vi "SaveData_Rf.vi"(8 "error in (no error)":errorcluster, 11 "Data In":T1) -> (0 "error out":errorcluster, 3 "Data Out":T1)   [LabVIEW 2014]
uses:
  controls/Data.ctl
  <vilib>/Utility/file.llb/Write To Spreadsheet File (string).vi
panel:
  # "日期"
  # "機種名稱"
  # "機種代號"
  # "商品條碼"
  # "台"
  # "OK"
  # "NG"
  # "台"
  # "總計"
  # "台"
  # "日期"
  # "機種名稱"
  # "機種代號"
  # "商品條碼"
  # "台"
  # "OK"
  # "NG"
  # "台"
  # "總計"
  # "台"
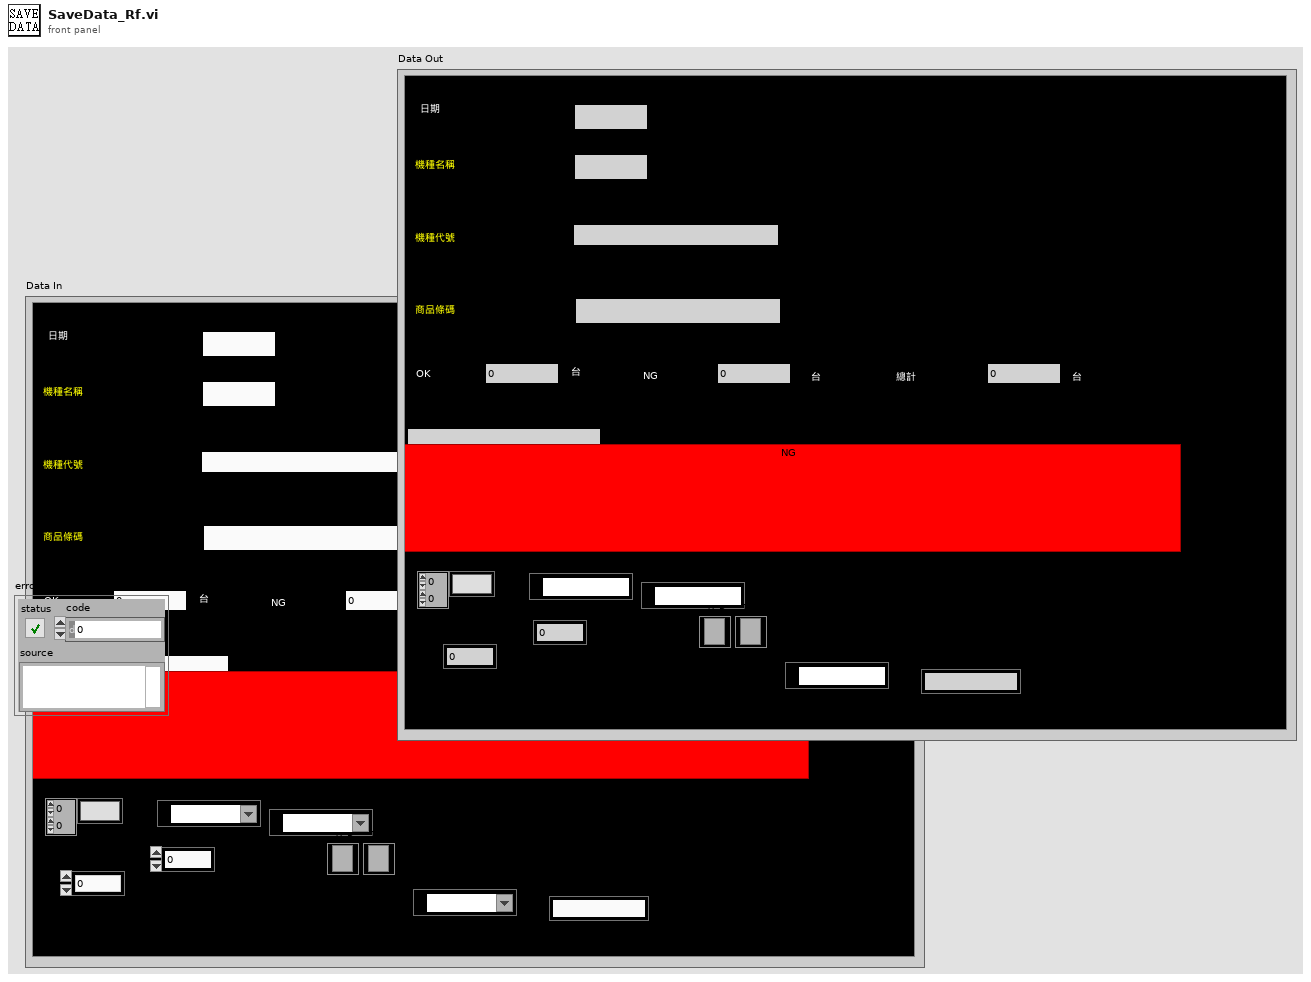
[diagram p1: front panel]
types:
  T1 = typedef "Data.ctl" = cluster{"Date":string, "BarCode1":string, "BarCode2":string, "BarCode3":string, "Message":string, "OK Count":u16, "NG Count":u16, "Total Count":u16, "ModelData":string[][], "OK&NG":bool, "COM1":refnum<visa-resource-name>, "COM2":refnum<visa-resource-name>, "IO":i32, "Time":u32, "TCP":refnum<k5>, "TCP 2":refnum<k5>, "COM3":refnum<visa-resource-name>, "CheckPars":string}
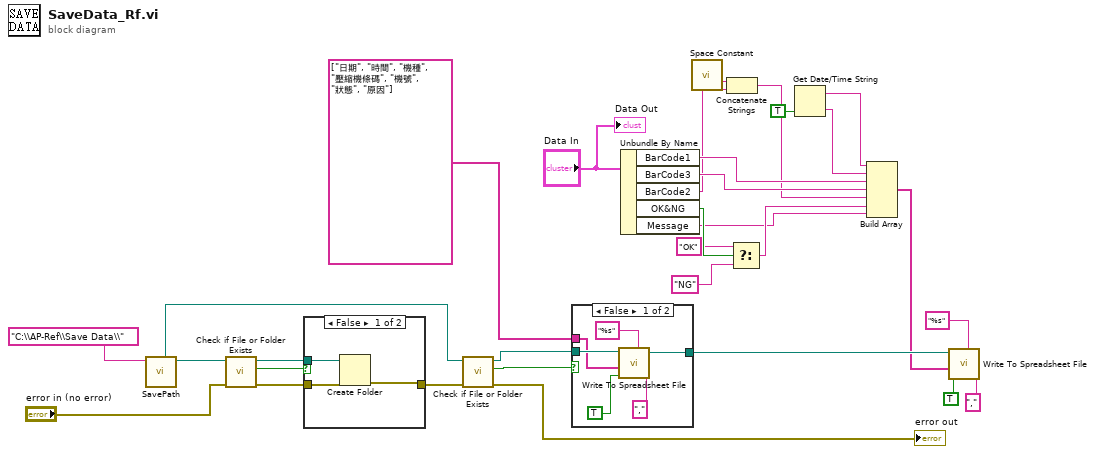
[diagram p0: block diagram]
diagram:
  n1 = call "SavePath.vi"("Path In"="C:\\AP-Ref\\Save Data\\") -> ("Folder Path"=w28:path, "File Path"=w26:path)  [unwired: 9 in]
  n2 = call <vilib>:"Check if File or Folder Exists.vi"("error in (no error)"="error in (no error)", "path"=w28) -> ("error out"=w25:errorcluster, "file or folder exists?"=w27:bool, "dup path"=w23:path)  [unwired: 7 in]
  n3 = case shown="False" w27 {
    tunnel: w25 -> [w33 w35]
    tunnel: [w32 w35] -> w24
    tunnel: w23 -> [w34 _]
    frame False {
      n4 = Create Folder(path (use dialog)=w34, error in=w33) -> (error out=w32:errorcluster)  [unwired: 1 in, 2 out]
    }
    frame True {
    }
  }
  n5 = call <vilib>:"Check if File or Folder Exists.vi"("error in (no error)"=w24, "path"=w26) -> ("error out"=→"error out":errorcluster, "file or folder exists?"=w21:bool, "dup path"=w22:path)  [unwired: 7 in]
  n6 = case shown="False" w21 {
    tunnel: w22 -> [w41 w42]
    tunnel: [w39 w42] -> w15
    tunnel: string[] ["日期", "時間", "機種", "壓縮機條碼", "機號", "狀態", "原因"] -> [w36 _]
    frame False {
      n7 = call-poly <vilib>:"Write To Spreadsheet File.vi"("delimiter (\\t)"="," ("delimiter (\\t)"), "format (%s)"="%s" ("format (%.3f)"), "append to file? (new file:F)"=TRUE, "1D data"=w36, "file path (dialog if empty)"=w41) -> ("new file path (Not A Path if cancelled)"=w39:path)  [unwired: 3 in]
    }
    frame True {
    }
  }
  n8 = Unbundle By Name("Data In") -> ("BarCode1"=w17:string, "BarCode3"=w7:string, "BarCode2"=w6:string, "OK&NG"=w20:bool, "Message"=w10:string)
  n9 = call <vilib>:"Space Constant.vi"() -> ("String"=w9:string)
  n10 = Concatenate Strings(w9, w6) -> (w5:string)
  n11 = Select(t="OK", s=w20, f="NG") -> (s? t:f=w16:string)
  n12 = Get Date/Time String(want seconds? (F)=TRUE) -> (date string=w3:string, time string=w4:string)  [unwired: 2 in]
  n13 = Build Array(w3, w4, w17, w7, w5, w16, w10) -> (w14:string[])
  n14 = call-poly <vilib>:"Write To Spreadsheet File.vi"("delimiter (\\t)"="," ("delimiter (\\t)"), "format (%s)"="%s", "append to file? (new file:F)"=TRUE, "1D data"=w14, "file path (dialog if empty)"=w15) -> ()  [unwired: 3 in, 1 out]
  "Data Out" <- "Data In"
